vi "Send buffered incidents.vi"(9 "Comms data":T1) -> (2 "Unsent":refnum<class "Incident.lvclass">[](array[class]))   [LabVIEW 2018]
uses:
  comms data.ctl
  Chris VIs/Incident logger/Incidents/Incident.lvclass
  <resource>/objmgr/ni.dex.rc
panel:
  out "Available Elements for Writing":i32
  out "incident buffer":string[][](array[string])
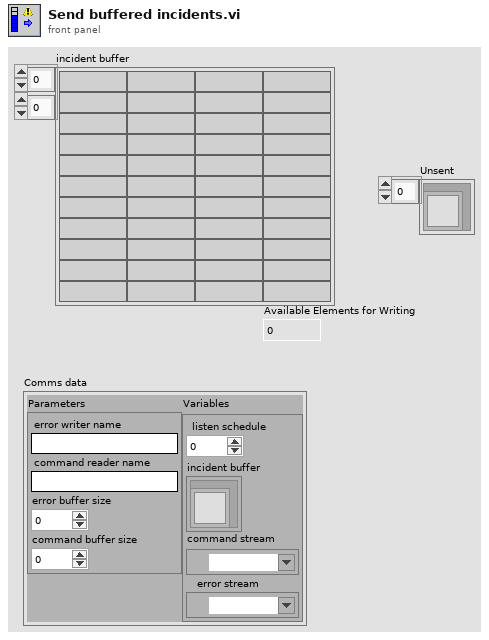
[diagram p1: front panel]
types:
  T1 = typedef "comms data.ctl" = cluster{"Parameters":cluster{"error writer name":string, "command reader name":string, "error buffer size":i32, "command buffer size":i32}, "Variables":cluster{"listen schedule":u32, "incident buffer":refnum<class "Incident.lvclass">[], "command stream":refnum<k21>, "error stream":refnum<k21>}}
  T2 = cluster{"type":string, "Time Stamp":timestamp, "Location":cluster{"Target":string, "Loop":string, "Code":string}, "Description":string, "error constant":errorcluster}
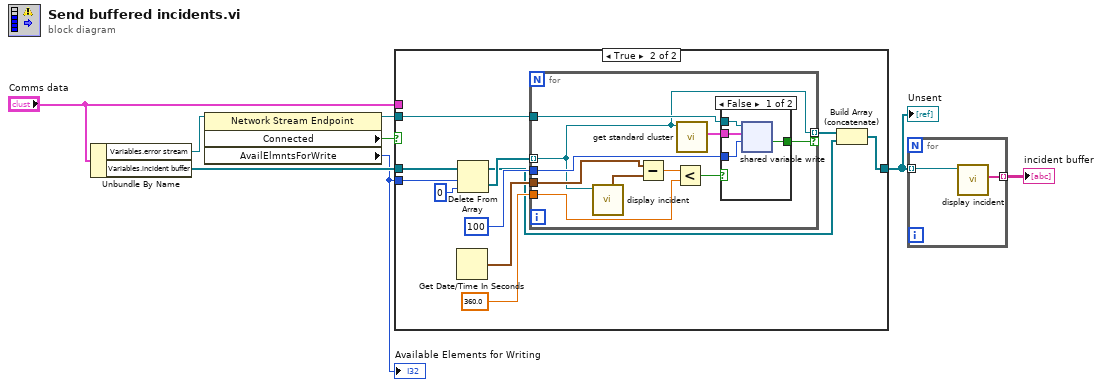
[diagram p0: block diagram]
diagram:
  n1 = Unbundle By Name("Comms data") -> ("Variables.error stream"=w7:refnum<k21>, "Variables.incident buffer"=w8:refnum<class "Incident.lvclass">[])
  n2 = property class="Network Stream Endpoint"(reference=w7) -> (reference out=w6:refnum<k21>, "Connected"=w5:bool, "AvailElmntsForWrite"=w1:i32)  [unwired: 1 in, 1 out]
  "Available Elements for Writing" <- w1
  n3 = case shown="True" w5 {
    tunnel: w8 -> [w9 w16]
    tunnel: w6 -> [_ w18]
    tunnel: "Comms data" -> [_ _]
    tunnel: [w9 w10] -> w3
    tunnel: w1 -> [_ w14]
    frame False {
    }
    frame True {
      n4 = Get Date/Time In Seconds() -> (seconds since 1Jan1904=w20:timestamp)
      n5 = Delete From Array(array=w16, length=w14, index=0 ("length")) -> (deleted portion=w13:refnum<class "Incident.lvclass">[], array with subset deleted=w11:refnum<class "Incident.lvclass">[])
      n6 = for {
        tunnel: w13 -> [w22] mode=indexing
        tunnel: w20 -> [w30]
        tunnel: 360.0 ("y") -> [w28]
        tunnel: w18 -> [w26]
        tunnel: 100 ("timeout ms (-1)") -> [w25]
        tunnel: [w22] -> w12 mode=indexing if=w21
        n7 = call-dynamic "display incident.vi"("Incident in"=w22) -> ("Time Stamp"=w29:timestamp)  [unwired: 5 in, 5 out]
        n8 = Subtract(x=w30, y=w29) -> (x-y=w27:dbl)
        n9 = Less?(x=w27, y=w28) -> (x < y?=w23:bool)
        n10 = call-dynamic "get standard cluster.vi"("Incident"=w22) -> ("standard cluster"=w24:T2)  [unwired: 10 in]
        n11 = case shown="False" w23 {
          tunnel: w26 -> [w34 _]
          tunnel: w25 -> [w33 _]
          tunnel: w24 -> [w32 _]
          tunnel: [w31 _] -> w21
          frame False {
            n12 = shared-variable-write(w34, w32, w33) -> (w31:bool)  [unwired: 1 in, 2 out]
          }
          frame True {
          }
        }
      }
      n13 = Build Array (concatenate)(w12, w11) -> (w10:refnum<class "Incident.lvclass">[])
    }
  }
  "Unsent" <- w3
  n14 = for {
    tunnel: w3 -> [w36] mode=indexing
    tunnel: [w35] -> w2 mode=indexing
    n15 = call-dynamic "display incident.vi"("Incident in"=w36) -> ("table string"=w35:string[])  [unwired: 5 in, 5 out]
  }
  "incident buffer" <- w2
